vi "Send Start Long Running Process.vi"(7 "Message Priority (Normal)":T1=enum."Normal", 8 "error in (no error)":errorcluster, 11 "Message Enqueuer":refnum<class "Message Enqueuer.lvclass">) -> (0 "error out":errorcluster, 2 "Future":refnum<class "Future.lvclass">, 3 "Message Enqueuer out":refnum<class "Message Enqueuer.lvclass">)   [LabVIEW 2017, in "Actor Example.lvlib" / "Start Long Running Process Msg.lvclass"]
doc: "This VI sends the message to an actor."
uses:
  Start Long Running Process Msg.lvclass
  <vilib>/ActorFramework/Message Enqueuer/Message Enqueuer.lvclass
  <vilib>/ActorFramework/Message Enqueuer/Message Priority.ctl
  Promise Future/Future/Future.lvclass
  C:/Program Files (x86)/National Instruments/LabVIEW 2017/vi.lib/ActorFramework/Message/Message.lvclass
  Start Long Running Process Msg.lvclass/Start Long Running Process Msg.ctl
  <vilib>/ActorFramework/Message Enqueuer/Message Enqueuer.lvclass/Message Enqueuer.ctl
  <vilib>/ActorFramework/Message Priority Queue/Priority Enqueue.vi
  Promise Future/Promise/Promise.lvclass
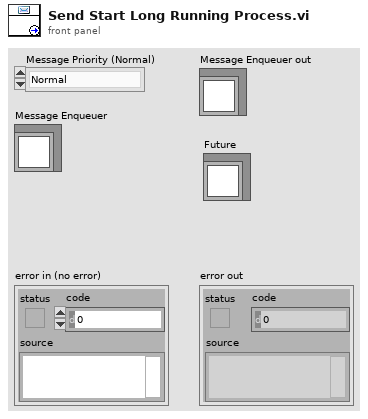
[diagram p1: front panel]
types:
  T1 = typedef "Actor Framework.lvlib/Message Enqueuer.lvclass/Message Priority.ctl" = enum16{"Low", "Normal", "High"}
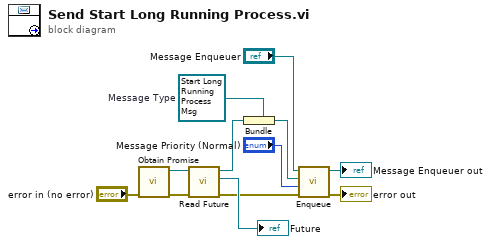
[diagram p0: block diagram]
diagram:
  w7 = refnum<class "Start Long Running Process Msg.lvclass"> refnum  # Message Type
  n1 = call "Obtain Promise.vi"("error in (no error)"="error in (no error)") -> ("error out"=w2:errorcluster, "Promise out"=w5:refnum<class "Promise.lvclass">)  [unwired: 8 in, 1 out]
  n2 = call "Read Future.vi"("error in (no error)"=w2, "Promise in"=w5) -> ("error out"=w1:errorcluster, "Future"=→"Future":refnum<class "Future.lvclass">, "Promise out"=w4:refnum<class "Promise.lvclass">)  [unwired: 7 in]
  n3 = Bundle(cluster=w7, w4) -> (w8:refnum<class "Start Long Running Process Msg.lvclass">)
  n4 = call <vilib>:"Enqueue.vi"("error in (no error)"=w1, "Message Priority (Normal)"="Message Priority (Normal)", "Message"=w8, "Message Enqueuer in"="Message Enqueuer") -> ("error out"=→"error out":errorcluster, "Message Enqueuer out"=→"Message Enqueuer out":refnum<class "Message Enqueuer.lvclass">)  [unwired: 6 in]
